vi "setLaserWavelength.vi"(3 "error in (no error)":errorcluster, 4 "End Wavelength (nm)":dbl format="%.2f", 5 "Start Wavelength (nm)":dbl format="%.2f") -> (0 "error out":errorcluster, 2 "Return Code":i32)   [LabVIEW 2024]
uses:
  Program Files (x86)/Luna Technologies/OVA 5000 v5.14.2/data/OVA32.dll
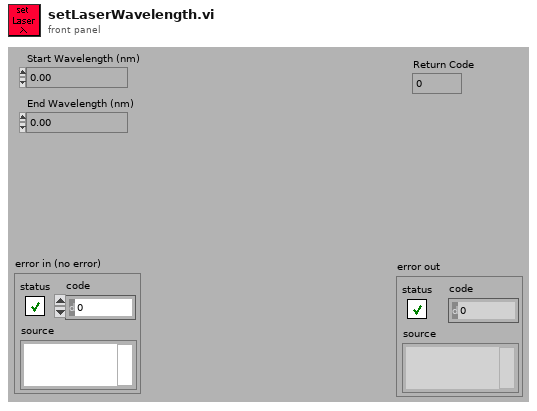
[diagram p1: front panel]
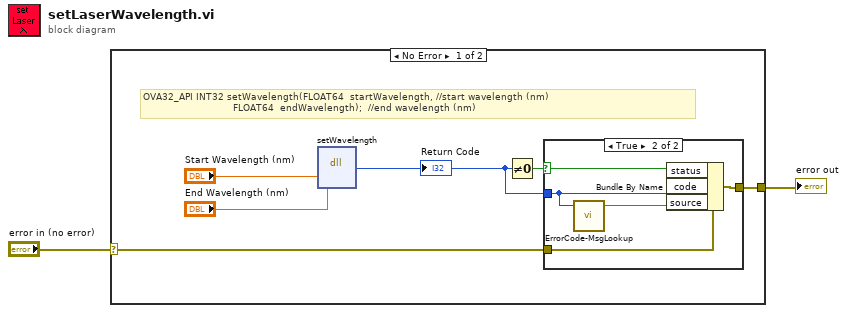
[diagram p0: block diagram]
diagram:
  n1 = case shown="No Error" "error in (no error)" {
    selector: "error in (no error)" -> [w4 w15]
    tunnel: [w3 w15] -> w1
    frame No Error {
      # "OVA32_API INT32 setWavelength(FLOAT64  startWavelength, //start wavelength (nm)\n                              FLOAT64  endWavelength);  //end wavelength (nm)"
      n2 = dll-call lib="C:/Program Files (x86)/Luna Technologies/OVA 5000 v5.14.2/data/OVA32.dll" fn="setWavelength"("startWavelength"="Start Wavelength (nm)", "endWavelength"="End Wavelength (nm)") -> (w6:i32)  [unwired: 5 in, 2 out]
      "Return Code" <- w6
      n3 = Not Equal To 0?(x=w6) -> (x != 0?=w8:bool)
      n4 = case shown="True" w8 {
        selector: w8 -> [_ w12]
        tunnel: w6 -> [_ w11]
        tunnel: w4 -> [w9 w14]
        tunnel: [w9 w13] -> w3
        frame False {
        }
        frame True {
          n5 = call "ErrorCode-MsgLookup.vi"("DLL Return Code"=w11) -> ("Error String"=w10:string)  [unwired: 2 in, 2 out]
          n6 = Bundle By Name(cluster=w14, "status"=w12, "code"=w11, "source"=w10) -> (w13:errorcluster)
        }
      }
    }
    frame Error {
    }
  }
  "error out" <- w1
